vi "Get 5-Rayleigh Parameters(SubVI).vi"(6 "Flow Peak Amp.":dbl, 8 "T_Flow Start (s)":dbl, 9 "T_Flow Peak (s)":dbl, 10 "T_Ejection period (s)":dbl, 11 "Pressure (mmHg)":waveform(dbl)) -> (3 "Optimised Parameter":dbl[](array[numeric]))   [LabVIEW 2017]
uses:
  72fe1329-4430-4fd7-86c8-dfab2f7b2d2e.vi
  5c84d562-1cd3-438d-9587-7d7d9e0fcbf7.vi
panel:
  out "sorted 2D array":dbl[][](array[numeric])
  out "x-1":i32
  out "sorted array of params":dbl[][](array[numeric])
  out "Error Checks":dbl[][](array[numeric])
  out "Parameters":dbl[][](array[numeric])
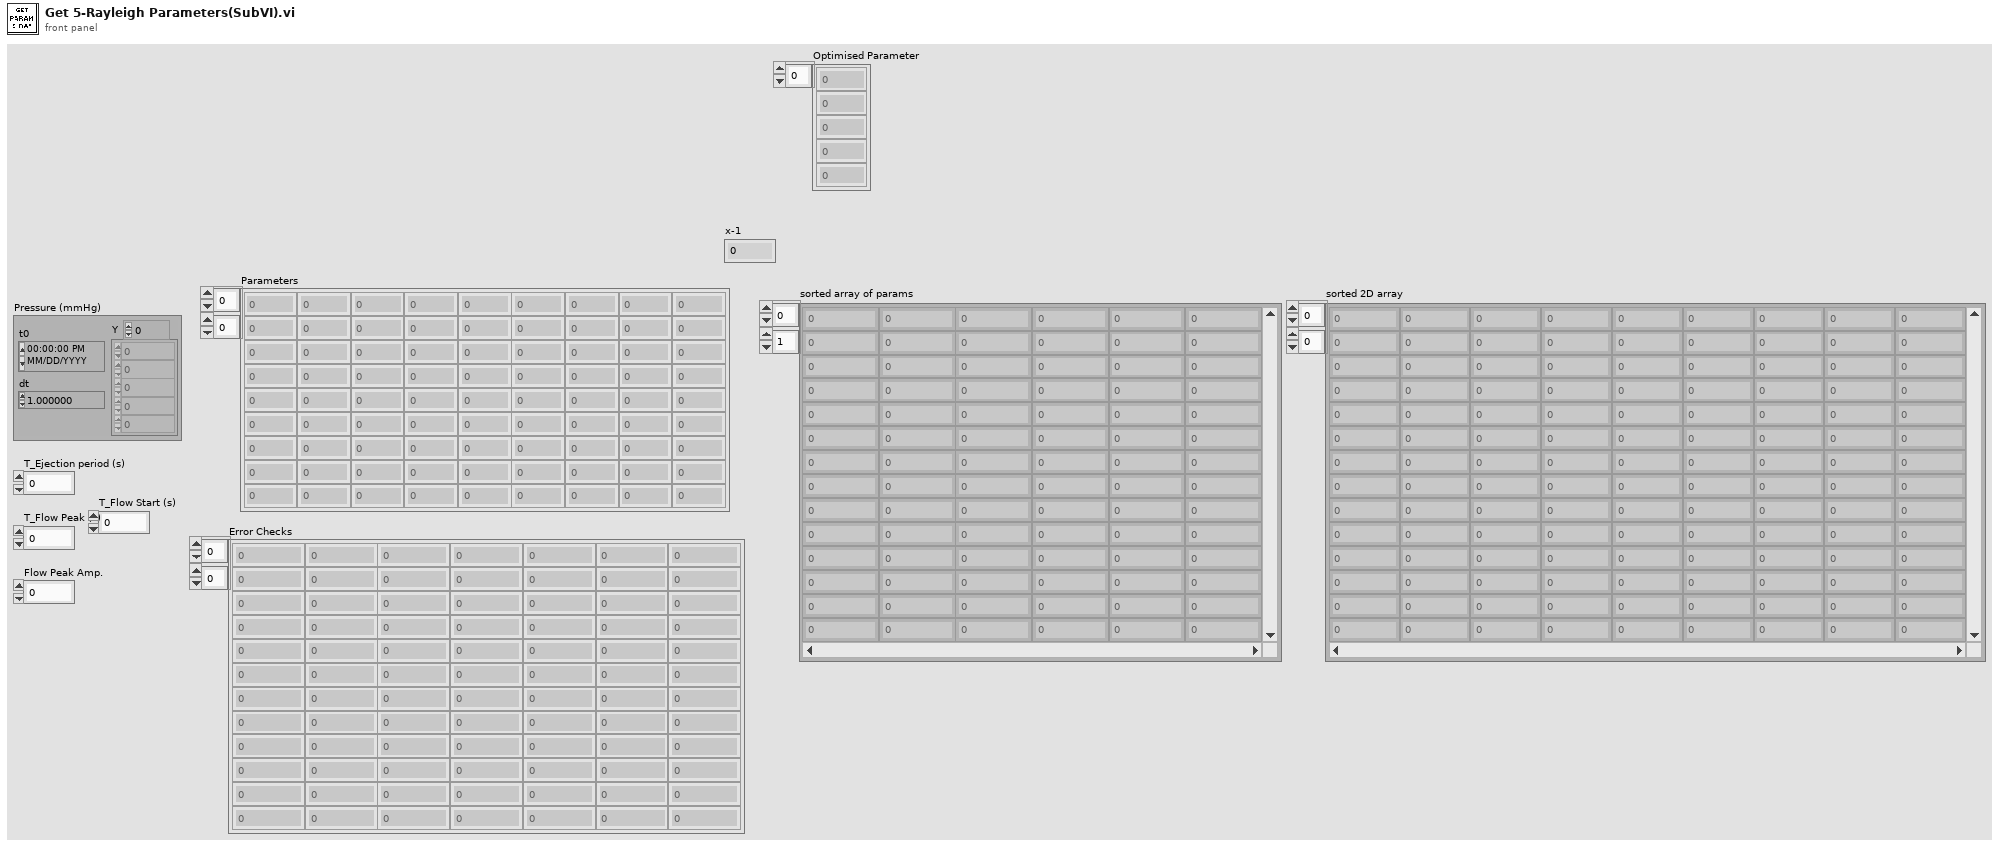
[diagram p1: front panel]
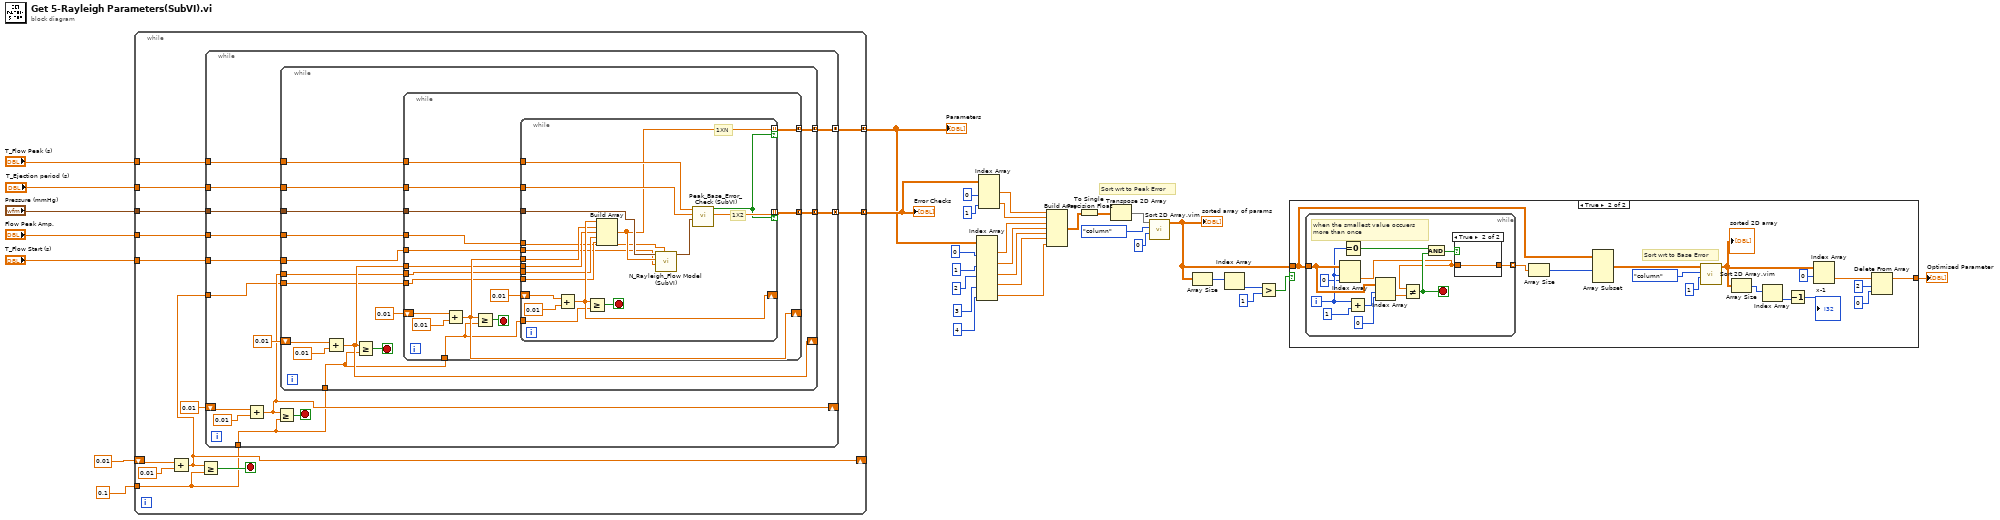
[diagram p0: block diagram]
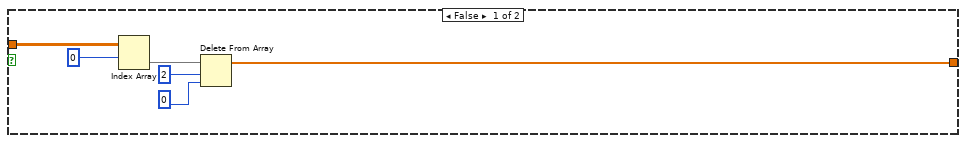
[diagram p2: hidden frame]
diagram:
  # "Sort wrt to Peak Error"
  n1 = while {
    tunnel: "Pressure (mmHg)" -> [w47]
    tunnel: "Flow Peak Amp." -> [w46]
    tunnel: "T_Ejection period (s)" -> [w45]
    tunnel: "T_Flow Peak (s)" -> [w44]
    tunnel: [w43] -> w24 mode=concatenating
    tunnel: [w42] -> w19 mode=concatenating
    tunnel: "T_Flow Start (s)" -> [w41]
    shift-right: [w36] -> _
    shift-left: 0.01 ("start") -> [w38]
    tunnel: 0.1 ("start") -> [w35]
    stop <- w37 stop-if-true
    n2 = Add(x=w38, y=0.01 ("start")) -> (x+y=w36:dbl)
    n3 = Greater Or Equal?(x=w36, y=w35) -> (x >= y?=w37:bool)
    n4 = while {
      tunnel: w47 -> [w61]
      tunnel: w46 -> [w60]
      tunnel: w45 -> [w59]
      tunnel: w44 -> [w58]
      tunnel: [w57] -> w43 mode=concatenating
      tunnel: [w56] -> w42 mode=concatenating
      tunnel: w41 -> [w55]
      shift-right: [w50] -> _
      shift-left: 0.01 ("start") -> [w52]
      tunnel: w36 -> [w49]
      tunnel: w35 -> [w48]
      stop <- w51 stop-if-true
      n5 = Add(x=w52, y=0.01 ("start")) -> (x+y=w50:dbl)
      n6 = Greater Or Equal?(x=w50, y=w48) -> (x >= y?=w51:bool)
      n7 = while {
        tunnel: w61 -> [w76]
        tunnel: w60 -> [w75]
        tunnel: w59 -> [w73]
        tunnel: w58 -> [w72]
        tunnel: [w71] -> w57 mode=concatenating
        tunnel: [w70] -> w56 mode=concatenating
        tunnel: w55 -> [w69]
        shift-right: [w65] -> _
        shift-left: 0.01 ("start") -> [w67]
        tunnel: w50 -> [w64]
        tunnel: w49 -> [w63]
        tunnel: w48 -> [w62]
        stop <- w66 stop-if-true
        n8 = Add(x=w67, y=0.01 ("start")) -> (x+y=w65:dbl)
        n9 = Greater Or Equal?(x=w65, y=w62) -> (x >= y?=w66:bool)
        n10 = while {
          tunnel: w76 -> [w92]
          tunnel: w75 -> [w91]
          shift-right: [w87] -> _
          shift-left: 0.01 ("start") -> [w89]
          tunnel: w73 -> [w85]
          tunnel: w72 -> [w84]
          tunnel: [w83] -> w70 mode=concatenating
          tunnel: [w82] -> w71 mode=concatenating
          tunnel: w69 -> [w81]
          tunnel: w65 -> [w80]
          tunnel: w64 -> [w79]
          tunnel: w63 -> [w78]
          tunnel: w62 -> [w77]
          stop <- w88 stop-if-true
          n11 = Add(x=w89, y=0.01 ("start")) -> (x+y=w87:dbl)
          n12 = Greater Or Equal?(x=w87, y=w77) -> (x >= y?=w88:bool)
          n13 = while {
            tunnel: w92 -> [w97]
            tunnel: w91 -> [w94]
            tunnel: w87 -> [w102]
            shift-right: [w103] -> _
            shift-left: 0.01 ("start") -> [w109]
            tunnel: w85 -> [w107]
            tunnel: w84 -> [w106]
            tunnel: [w96] -> w83 mode=indexing if=w104
            tunnel: [w105] -> w82 mode=indexing if=w104
            tunnel: w81 -> [w95]
            tunnel: w80 -> [w101]
            tunnel: w79 -> [w100]
            tunnel: w78 -> [w99]
            tunnel: w77 -> [w98]
            stop <- w108 stop-if-true
            # "1X2"
            # "1XN"
            n14 = Add(x=w109, y=0.01 ("start")) -> (x+y=w103:dbl)
            n15 = Greater Or Equal?(x=w103, y=w98) -> (x >= y?=w108:bool)
            n16 = Build Array(w103, w102, w101, w100, w99) -> (w96:dbl[])
            n17 = call "N_Rayleigh_Flow Model (SubVI).vi"("PSQ (ml/s)"=w94, "T_Flow Start"=w95, "Parameters (1XN)"=w96, "Pressure (mmHg)"=w97) -> ("n-Rayleigh Model Flow"=w93:waveform(dbl))  [unwired: 4 in, 1 out]
            n18 = call "Peak_Base_Error_Check (SubVI).vi"("Model Flow"=w93, "T_Ejection Period (s)"=w107, "T_Flow Peak (s)"=w106) -> ("Error"=w105:dbl[], "Logic"=w104:bool)  [unwired: 5 in, 2 out]
          }
        }
      }
    }
  }
  "Parameters" <- w19
  "Error Checks" <- w24
  n19 = Index Array(array=w19, index (col) #1=0 ("disabled index (col)"), index (col) #2=1 ("index (col)"), index (col) #3=2 ("index (col)"), index (col) #4=3 ("index (col)"), index (col) #5=4 ("index (col)")) -> (element #1=w21:dbl[], element #2=w20:dbl[], element #3=w7:dbl[], element #4=w5:dbl[], element #5=w2:dbl[])  [unwired: 5 in]
  n20 = Index Array(array=w24, index (col) #1=0 ("disabled index (col)"), index (col) #2=1 ("index (col)")) -> (element #1=w23:dbl[], element #2=w22:dbl[])  [unwired: 2 in]
  n21 = Build Array(w23, w22, w21, w20, w7, w5, w2) -> (w10:dbl[][])
  n22 = To Single Precision Float(number=w10) -> (single precision float=w11:sgl[][])
  n23 = Transpose 2D Array(2D array=w11) -> (transposed array=w18:sgl[][])
  n24 = call "Sort 2D Array.vim"("index"=0, "dimension to index (column)"=enum16{"column", "row"}."column", "2D array"=w18) -> ("sorted 2D array"=w12:sgl[][])  [unwired: 7 in, 1 out]
  "sorted array of params" <- w12
  n25 = Array Size(array=w12) -> (size(s)=w16:i32[])
  n26 = Index Array(array=w16) -> (element=w15:i32)  [unwired: 1 in]
  n27 = Greater?(x=w15, y=1) -> (0:w14:bool)
  n28 = case shown="True" w14 {
    tunnel: w12 -> [w116 w120]
    tunnel: [w111 w119] -> w13
    frame False {
      n29 = Index Array(array=w116, index (row)=0) -> (element=w114:sgl[])  [unwired: 1 in]
      n30 = Delete From Array(array=w114, length=2, index=0) -> (array with subset deleted=w111:sgl[])  [unwired: 1 out]
    }
    frame True {
      # "Sort wrt to Base Error"
      n31 = while {
        tunnel: w120 -> [w141]
        tunnel: [w138] -> w121 mode=indexing
        i -> [w140]
        stop <- w134 stop-if-true
        # "when the smallest value occuers \nmore than once"
        n32 = Index Array(array=w141, index (row)=w140, index (col)=0 ("disabled index (col)")) -> (element=w133:sgl)
        n33 = Equal To 0?(x=w140) -> (x = 0?=w139:bool)
        n34 = Add(x=w140, y=1) -> (x+y=w142:i32)
        n35 = Index Array(array=w141, index (row)=w142, index (col)=0 ("disabled index (col)")) -> (element=w132:sgl)
        n36 = Not Equal?(x=w133, y=w132) -> (x != y?=w134:bool)
        n37 = And(x=w139, y=w134) -> (x .and. y?=w135:bool)
        n38 = case shown="True" w135 {
          tunnel: w133 -> [w144 w145]
          tunnel: [w144 w145] -> w138
          frame False {
          }
          frame True {
          }
        }
      }
      n39 = Array Size(array=w121) -> (size(s)=w118:i32)
      n40 = Array Subset(array=w120, length (row)=w118) -> (w126:sgl[][])  [unwired: 3 in]
      n41 = call "Sort 2D Array.vim"("index"=1, "dimension to index (column)"=enum16{"column", "row"}."column", "2D array"=w126) -> ("sorted 2D array"=w127:sgl[][])  [unwired: 7 in, 1 out]
      "sorted 2D array" <- w127
      n42 = Array Size(array=w127) -> (size(s)=w128:i32[])
      n43 = Index Array(array=w128) -> (element=w129:i32)  [unwired: 1 in]
      n44 = Decrement(x=w129) -> (x-1=→"x-1":i32)
      n45 = Index Array(array=w127, index (row)=0) -> (element=w131:sgl[])  [unwired: 1 in]
      n46 = Delete From Array(array=w131, length=2, index=0) -> (array with subset deleted=w119:sgl[])  [unwired: 1 out]
    }
  }
  "Optimised Parameter" <- w13
